vi "Controller 1.vi"() -> (0 "Buttons":T2, 1 "Axes":T1)   [LabVIEW 2013]
uses:
  <vilib>/Rock Robotics/WPI/Joystick/WPI_JoystickGetSetRefNum.vi
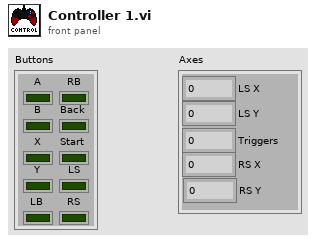
[diagram p1: front panel]
types:
  T1 = cluster{"LS X":dbl, "LS Y":dbl, "Triggers":dbl, "RS X":dbl, "RS Y":dbl}
  T2 = cluster{"A":bool, "B":bool, "X":bool, "Y":bool, "LB":bool, "RB":bool, "Back":bool, "Start":bool, "LS":bool, "RS":bool}
  T3 = typedef "WPI_JoystickDevRef.ctl" = cluster{"Device":T4}
  T4 = typedef "WPI_JoystickDeviceEnum.ctl" = enum16{"USB 1", "USB 2", "USB 3", "USB 4", "Kinect 1", "Kinect 2"}
  T5 = typedef "WPI_JoystickButtonState.ctl" = cluster{"Button 1":bool, "Button 2":bool, "Button 3":bool, "Button 4":bool, "Button 5":bool, "Button 6":bool, "Button 7":bool, "Button 8":bool, "Button 9":bool, "Button 10":bool, "Button 11":bool, "Button 12":bool}
  T6 = cluster{"axis 1 (x)":dbl, "axis 2 (y)":dbl, "axis 3 (throttle)":dbl, "axis 4":dbl, "axis 5":dbl, "axis 6":dbl}
  T7 = cluster{"axis 1 (x)":dbl, "axis 2 (y)":dbl, "axis 3 (throttle)":dbl, "axis 4":dbl, "axis 5":dbl}
  T8 = cluster{"Button 1":bool, "Button 2":bool, "Button 3":bool, "Button 4":bool, "Button 5":bool, "Button 6":bool, "Button 7":bool, "Button 8":bool, "Button 9":bool, "Button 10":bool}
  T9 = cluster{"[0]":dbl, "[1]":dbl, "[2]":dbl, "[3]":dbl, "[4]":dbl}
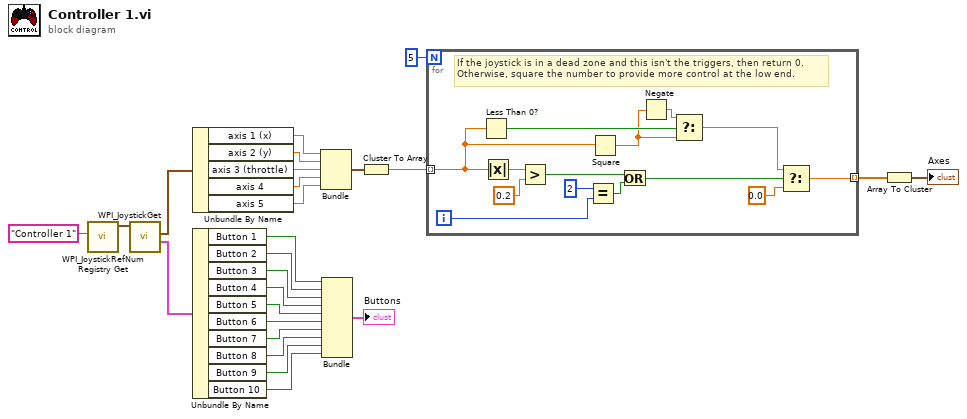
[diagram p0: block diagram]
diagram:
  n1 = call <vilib>:"WPI_JoystickRefNum Registry Get.vi"("refnum name"="Controller 1") -> ("JoystickDevRef"=w25:T3)  [unwired: 9 in, 1 out]
  n2 = call <vilib>:"WPI_JoystickGet.vi"("JoystickDevRef"=w25) -> ("Buttons"=w24:T5, "Axes"=w12:T6)  [unwired: 4 in, 1 out]
  n3 = Unbundle By Name(w12) -> ("axis 1 (x)"=w11:dbl, "axis 2 (y)"=w10:dbl, "axis 3 (throttle)"=w9:dbl, "axis 4"=w8:dbl, "axis 5"=w7:dbl)
  n4 = Unbundle By Name(w24) -> ("Button 1"=w23:bool, "Button 2"=w22:bool, "Button 3"=w21:bool, "Button 4"=w20:bool, "Button 5"=w19:bool, "Button 6"=w18:bool, "Button 7"=w17:bool, "Button 8"=w16:bool, "Button 9"=w15:bool, "Button 10"=w14:bool)
  n5 = Bundle("axis 1 (x)"=w11, "axis 2 (y)"=w10, "axis 3 (throttle)"=w9, "axis 4"=w8, "axis 5"=w7) -> (w5:T7)  [unwired: 1 in]
  n6 = Bundle("Button 1"=w23, "Button 2"=w22, "Button 3"=w21, "Button 4"=w20, "Button 5"=w19, "Button 6"=w18, "Button 7"=w17, "Button 8"=w16, "Button 9"=w15, "Button 10"=w14) -> (→"Buttons":T8)  [unwired: 1 in]
  n7 = Cluster To Array(cluster=w5) -> (array=w3:dbl[])
  n8 = for {
    N: 5 -> [_]
    tunnel: w3 -> [w33] mode=indexing
    tunnel: [w37] -> w2 mode=indexing
    i -> [w27]
    # "If the joystick is in a dead zone and this isn't the triggers, then return 0.\nOtherwise, square the number to provide more control at the low end."
    n9 = Less Than 0?(x=w33) -> (x < 0?=w35:bool)
    n10 = Absolute Value(x=w33) -> (abs(x)=w36:dbl)
    n11 = Greater?(x=w36, y=0.2) -> (0:w30:bool)
    n12 = Equal?(x=2, y=w27) -> (x = y?=w28:bool)
    n13 = Square(x=w33) -> (x^2=w32:dbl)
    n14 = Or(x=w30, y=w28) -> (x .or. y?=w29:bool)
    n15 = Negate(x=w32) -> (-x=w31:dbl)
    n16 = Select(t=w31, s=w35, f=w32) -> (s? t:f=w34:dbl)
    n17 = Select(t=w34, s=w29, f=0.0) -> (s? t:f=w37:dbl)
  }
  n18 = Array To Cluster(array=w2) -> (cluster=→"Axes":T9)
